vi "m1m3_getEvent_AppliedOffsetForces.vi"(8 "error in (no error)":errorcluster, 11 "logevent_AppliedOffsetForces_Ctl":T1) -> (0 "error out":errorcluster, 2 "function return":i32, 3 "logevent_AppliedOffsetForces_Ctl out":T1)   [LabVIEW 2016, in "SALLV_m1m3.lvlib"]
doc: "int m1m3_shm_getEvent_AppliedOffsetForcesLV(m1m3_logevent_AppliedOffsetForcesLV *logevent_AppliedOffsetForces_Ctl );"
uses:
  SALLV_m1m3.lvlib
  DataTypes/logevent_AppliedOffsetForces.ctl
  SALLV_m1m3.so
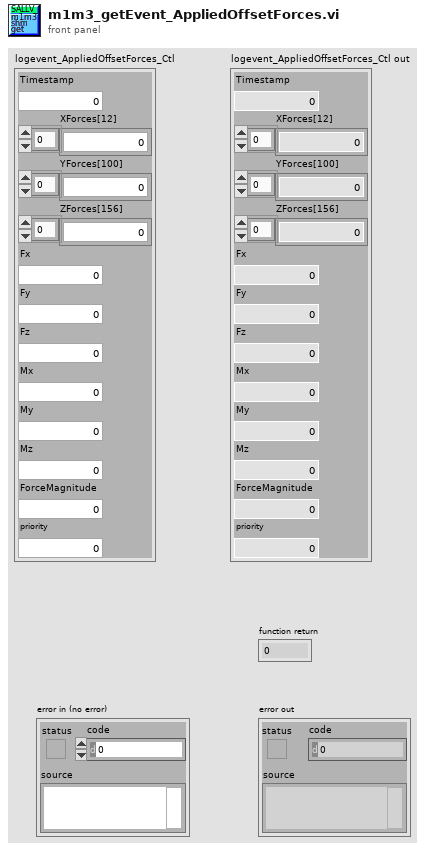
[diagram p1: front panel]
types:
  T1 = typedef "SALLV_m1m3.lvlib/logevent_AppliedOffsetForces.ctl" = cluster{"Timestamp":dbl, "XForces[12]":sgl[], "YForces[100]":sgl[], "ZForces[156]":sgl[], "Fx":sgl, "Fy":sgl, "Fz":sgl, "Mx":sgl, "My":sgl, "Mz":sgl, "ForceMagnitude":sgl, "priority":i32}
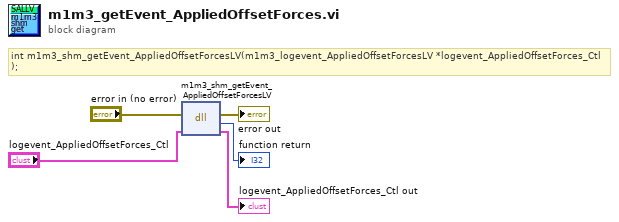
[diagram p0: block diagram]
diagram:
  # "int m1m3_shm_getEvent_AppliedOffsetForcesLV(m1m3_logevent_AppliedOffsetForcesLV *logevent_AppliedOffsetForces_Ctl );"
  n1 = dll-call lib="opt/CODE/SALLV_m1m3/SALLV_m1m3.*" fn="m1m3_shm_getEvent_AppliedOffsetForcesLV"(error in="error in (no error)", "logevent_AppliedOffsetForces_Ctl"="logevent_AppliedOffsetForces_Ctl") -> (error out=→"error out":errorcluster, →"function return":i32, "logevent_AppliedOffsetForces_Ctl"=→"logevent_AppliedOffsetForces_Ctl out":T1)  [unwired: 2 in, 1 out]
